vi "serialread.vi"() -> ()   [LabVIEW 2024]
uses:
  <vilib>/Native 3D Graph/xcontrol/3DPC_SurfacePlot.xctl
  <vilib>/Instr/_visa.llb/VISA Configure Serial Port (Instr).vi
  <vilib>/Native 3D Graph/classes/Base Datatype.lvclass
panel:
  out "3D Graph":refnum<class "Base Datatype.lvclass">[](xcontrol)
  out "Z":dbl
  out "Y":dbl
  out "X":dbl
  out "read buffer":string
  in  "Send":bool
  in  "CMD":string
  out "error out":errorcluster
  in  "stop":bool
  in  "VISA resource name":refnum<visa-resource-name>
  # "Test this VI by first running ASCII Streaming Instrument.vi.  You will need 2 serial ports that are connected via a NULL Modem cable."
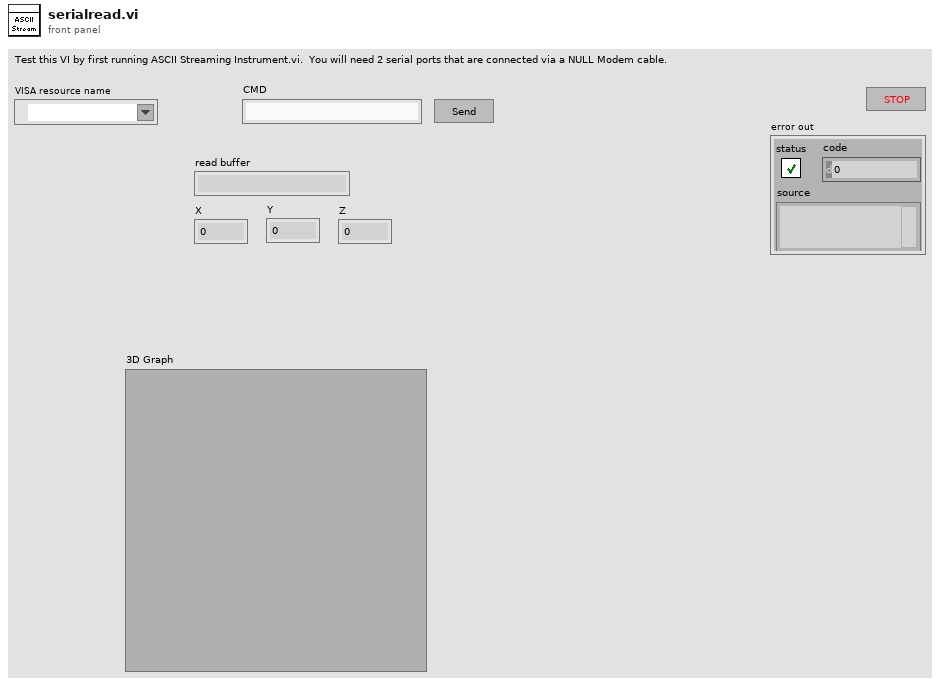
[diagram p1: front panel]
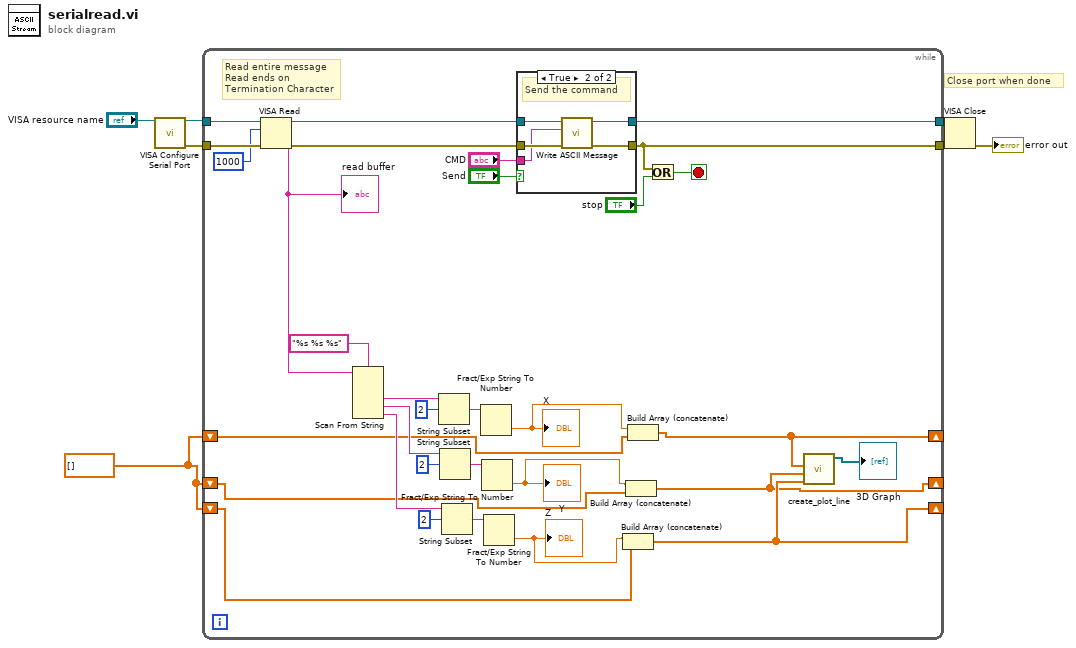
[diagram p0: block diagram]
diagram:
  w1 = dbl[] [] ("color vector")
  # "Close port when done"
  n1 = call-poly "VISA Configure Serial Port"("VISA resource name"="VISA resource name") -> ("VISA resource name out"=w2:refnum<visa-resource-name>, "error out"=w5:errorcluster)  [unwired: 13 in]
  n2 = while {
    tunnel: w5 -> [w39]
    tunnel: w2 -> [w36]
    tunnel: [w35] -> w3
    tunnel: [w38] -> w7
    shift-right: [w8] -> _
    shift-left: w1 -> [w14]
    shift-right: [w9] -> _
    shift-left: w1 -> [w13]
    shift-right: [w10] -> _
    shift-left: w1 -> [w12]
    stop <- w34 stop-if-true
    # "Read entire message\nRead ends on\nTermination Character"
    n3 = VISA Read(VISA resource name=w36, byte count=u32 1000, error in (no error)=w39) -> (VISA resource name out=w31:refnum<visa-resource-name>, read buffer=w28:string, error out=w37:errorcluster)  [unwired: 1 out]
    "read buffer" <- w28
    n4 = Scan From String(format string="%s %s %s", input string=w28) -> (output 1=w26:string, output 2=w18:string, output 3=w19:string)  [unwired: 5 in, 3 out]
    n5 = String Subset(string=w26, offset (0)=2) -> (substring=w24:string)  [unwired: 1 in]
    n6 = String Subset(string=w18, offset (0)=2) -> (substring=w22:string)  [unwired: 1 in]
    n7 = String Subset(string=w19, offset (0)=2) -> (substring=w20:string)  [unwired: 1 in]
    n8 = Fract/Exp String To Number(string=w24) -> (number=w17:dbl)  [unwired: 3 in, 1 out]
    "X" <- w17
    n9 = Fract/Exp String To Number(string=w22) -> (number=w15:dbl)  [unwired: 3 in, 1 out]
    "Y" <- w15
    n10 = Fract/Exp String To Number(string=w20) -> (number=w16:dbl)  [unwired: 3 in, 1 out]
    "Z" <- w16
    n11 = case shown="True" "Send" {
      tunnel: [w41 w46] -> w38
      tunnel: [w40 w44] -> w35
      tunnel: w37 -> [w41 w45]
      tunnel: w31 -> [w40 w43]
      tunnel: "CMD" -> [_ w42]
      frame False {
        # "Do nothing"
      }
      frame True {
        # "Send the command"
        n12 = call "Write ASCII Message.vi"("error in"=w45, "Message"=w42, "VISA resource in"=w43) -> ("error out"=w46:errorcluster, "VISA resource out"=w44:refnum<visa-resource-name>)  [unwired: 7 in]
      }
    }
    n13 = Build Array (concatenate)(w16, w12) -> (w10:dbl[])
    n14 = Build Array (concatenate)(w15, w13) -> (w9:dbl[])
    n15 = Build Array (concatenate)(w17, w14) -> (w8:dbl[])
    n16 = Or(x=w38, y="stop") -> (x .or. y?=w34:bool)
    n17 = call <vilib>:"create_plot_line.vi"("z vector"=w10, "y vector"=w9, "x vector"=w8) -> ("plots out"=→"3D Graph":refnum<class "Base Datatype.lvclass">[])  [unwired: 2 in, 6 out]
  }
  n18 = VISA Close(VISA resource name=w3, error in (no error)=w7) -> (error out=→"error out":errorcluster)
